vi "Test Timer API.vi"() -> ()   [LabVIEW 2018]
uses:
  Timer.lvclass
  Timer.lvclass/Timer.ctl
  Get Target Time Elapsed Event.vi
panel:
  out "error out":errorcluster
  out "Time Elapsed?":bool[](array[boolean])
  out "Timers":timestamp[](array[timestamp]) format="%^<%H:%M:%S>T"
  in  "Target Time (seconds)":dbl=10.0
  in  "Start Timer":bool caption="Open Door"
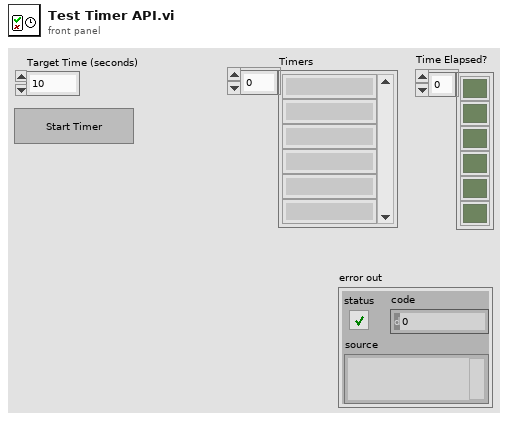
[diagram p1: front panel]
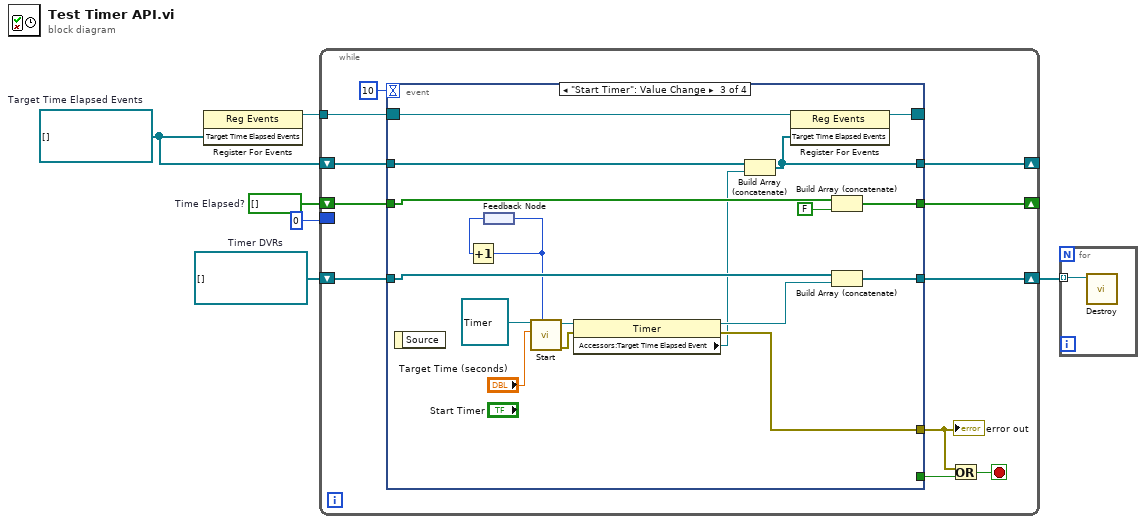
[diagram p0: block diagram]
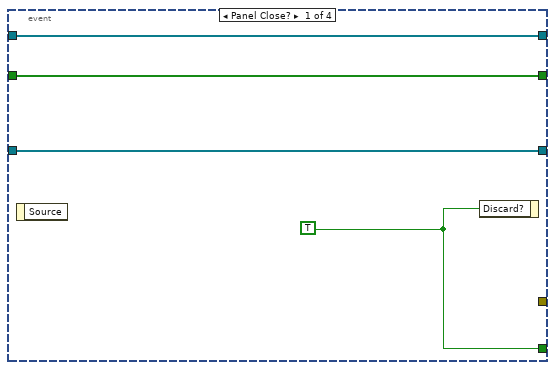
[diagram p2: hidden frame]
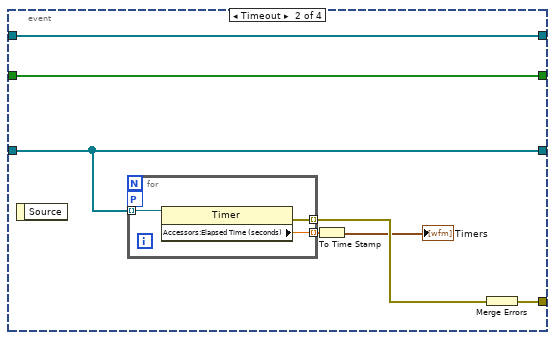
[diagram p3: hidden frame]
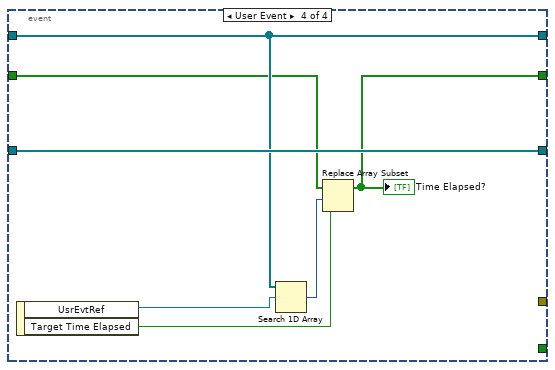
[diagram p4: hidden frame]
diagram:
  w3 = bool[] []  # Time Elapsed?
  w4 = refnum<user-event>[] []  # Target Time Elapsed Events
  w6 = refnum<data-value>[] []  # Timer DVRs
  n1 = register-events(w4) -> (reference out=w5:refnum<event-registration>)  [unwired: 2 in, 1 out]
  n2 = while {
    shift-right: [w15] -> w2
    shift-left: w6 -> [w16]
    tunnel: w5 -> [w13]
    shift-right: [w11] -> _
    shift-left: w4 -> [w12]
    shift-right: [w9] -> _
    shift-left: w3 -> [w10]
    border: 0 -> [_]
    stop <- w8 stop-if-true
    n3 = event shown="[2] \"Start Timer\": Value Change" {
      selector: w13 -> [_ _ w43 _]
      dyn-events: [_ _ w42 _] -> _
      timeout: 10 -> [_ _ _ _]
      tunnel: [w21 _ _ _] -> w17
      tunnel: w16 -> [w20 w27 w46 w56]
      tunnel: [w20 w27 w45 w56] -> w15
      tunnel: w12 -> [w19 w24 w41 w55]
      tunnel: [w19 w24 w40 w55] -> w11
      tunnel: w10 -> [w18 w23 w39 w53]
      tunnel: [w18 w23 w37 w50] -> w9
      tunnel: [_ w22 w48 _] -> w7
      event Panel Close? {
        w21 = TRUE ("Discard?")
        n4 = event-data() -> ()  [unwired: 1 in, 1 out]
        n5 = event-data("Discard?"=w21) -> ()  [unwired: 1 in, 1 out]
      }
      event Timeout {
        n6 = event-data() -> ()  [unwired: 1 in, 1 out]
        n7 = for {
          tunnel: w27 -> [w31] mode=indexing
          tunnel: [w30] -> w26 mode=indexing
          tunnel: [w29] -> w28 mode=indexing
          workers-P: _ -> [_]
          n8 = property class="Timer"(reference=w31) -> (error out=w29:errorcluster, "Accessors:Elapsed Time (seconds)"=w30:dbl)  [unwired: 1 in, 1 out]
        }
        n9 = To Time Stamp(1:w26) -> (0:→"Timers":timestamp[])
        n10 = Merge Errors(w28) -> (w22:errorcluster)
      }
      event "Start Timer": Value Change {
        n11 = event-data() -> ()  [unwired: 1 in, 1 out]
        n12 = feedback #1() -> (w33:i32)
        n13 = Increment(x=w33) -> (x+1=w32:i32)
        n14 = feedback-in #1(w32) -> ()
        n15 = call-dynamic "Start.vi"("Timer ID"=w32, "Target Time (seconds)"="Target Time (seconds)", "Timer in"=refnum<class "Timer.lvclass"> refnum ("Timer.lvclass")) -> ("error out"=w34:errorcluster, "Timer DVR"=w36:refnum<data-value>)  [unwired: 7 in]
        n16 = property class="Timer"(reference=w36, error in=w34) -> (reference out=w49:refnum<data-value>, error out=w48:errorcluster, "Accessors:Target Time Elapsed Event"=w35:refnum<user-event>)
        n17 = Build Array (concatenate)(w41, w35) -> (w40:refnum<user-event>[])
        n18 = register-events(reference=w43, w40) -> (reference out=w42:refnum<event-registration>)  [unwired: 1 in, 1 out]
        n19 = Build Array (concatenate)(w39, FALSE ("Boolean")) -> (w37:bool[])
        n20 = Build Array (concatenate)(w46, w49) -> (w45:refnum<data-value>[])
      }
      event User Event {
        n21 = event-data() -> ("UsrEvtRef"=w54:refnum<user-event>, "Target Time Elapsed"=w51:bool)  [unwired: 1 in]
        n22 = Search 1D Array(1D array=w55, element=w54) -> (index of element=w52:i32)  [unwired: 1 in]
        n23 = Replace Array Subset(array=w53, new element=w51, index=w52) -> (w50:bool[])
        "Time Elapsed?" <- w50
      }
    }
    "error out" <- w7
    n24 = Or(x=w7, y=w17) -> (x .or. y?=w8:bool)
  }
  n25 = for {
    tunnel: w2 -> [w57] mode=indexing
    n26 = call "Destroy.vi"("Timer DVR"=w57) -> ()  [unwired: 10 in, 1 out]
  }
